vi "locker-lock.vi"(8 "error in (no error)":errorcluster, 11 "queue":refnum<queue>) -> (0 "error out":errorcluster, 3 "locker(dup)":refnum<queue>)   [LabVIEW 2017]
doc: "Blocks until the locker is free and then takes it. Every locker-lock must be paired with a locker-unlock."
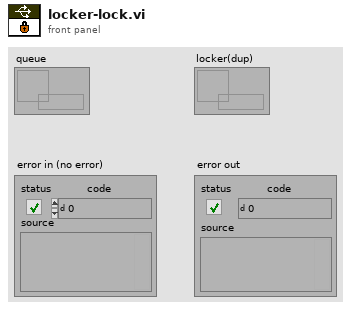
[diagram p1: front panel]
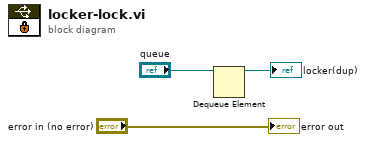
[diagram p0: block diagram]
diagram:
  n1 = Dequeue Element(queue="queue") -> (queue out=→"locker(dup)":refnum<queue>)  [unwired: 2 in, 3 out]
  "error out" <- "error in (no error)"
